vi "Cuadro de Texto.vi"(2 "Numeric":dbl, 3 "Read":refnum<k21>, 4 "Write":refnum<k21>, 5 "ECU TYPE":u16(ring) items=["LSMD", "LSMP", "LSMRL", "LSMRR"]) -> (0 "Write out":refnum<k21>, 1 "Read out":refnum<k21>)   [LabVIEW 2023]
panel:
  in  "OK":bool
  out "String":string
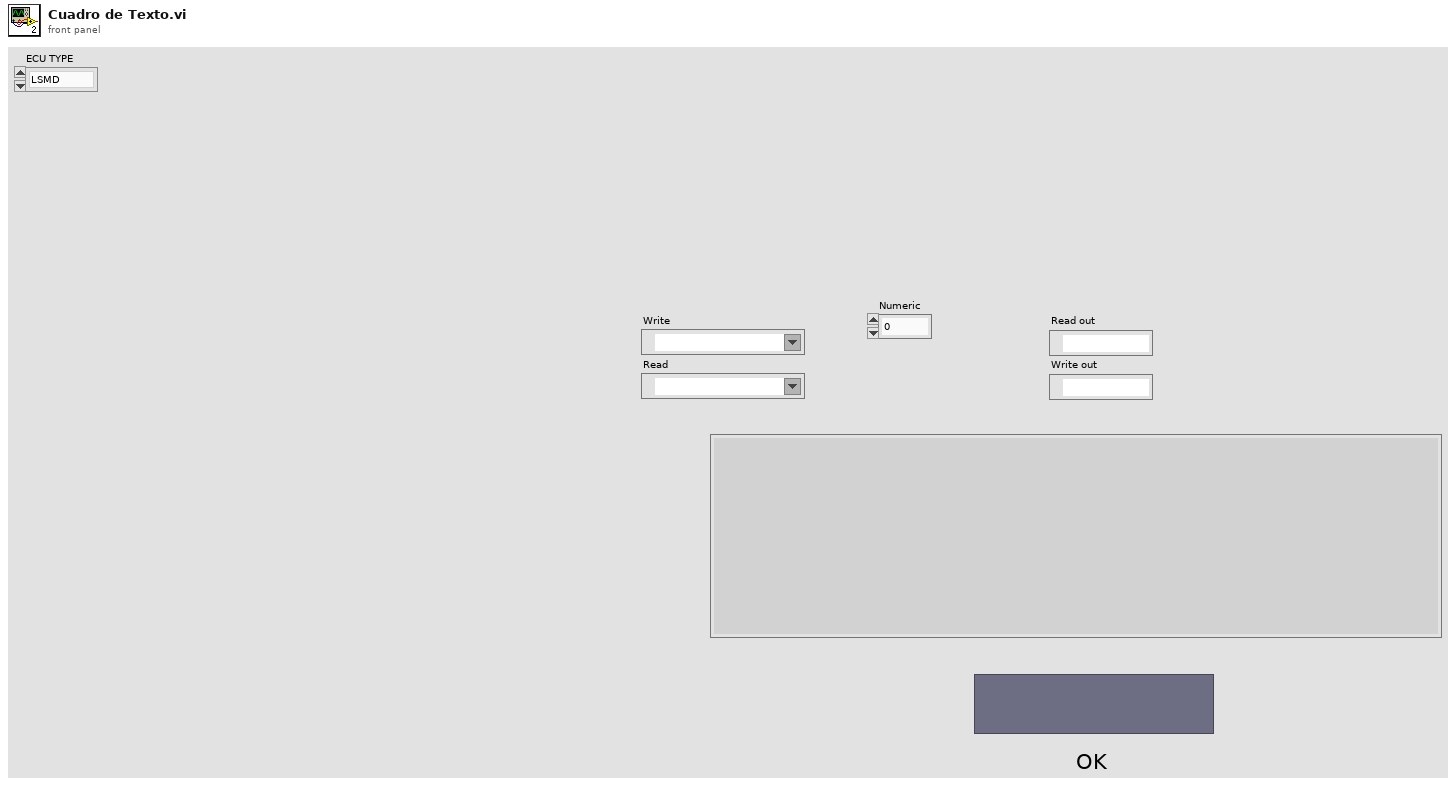
[diagram p1: front panel]
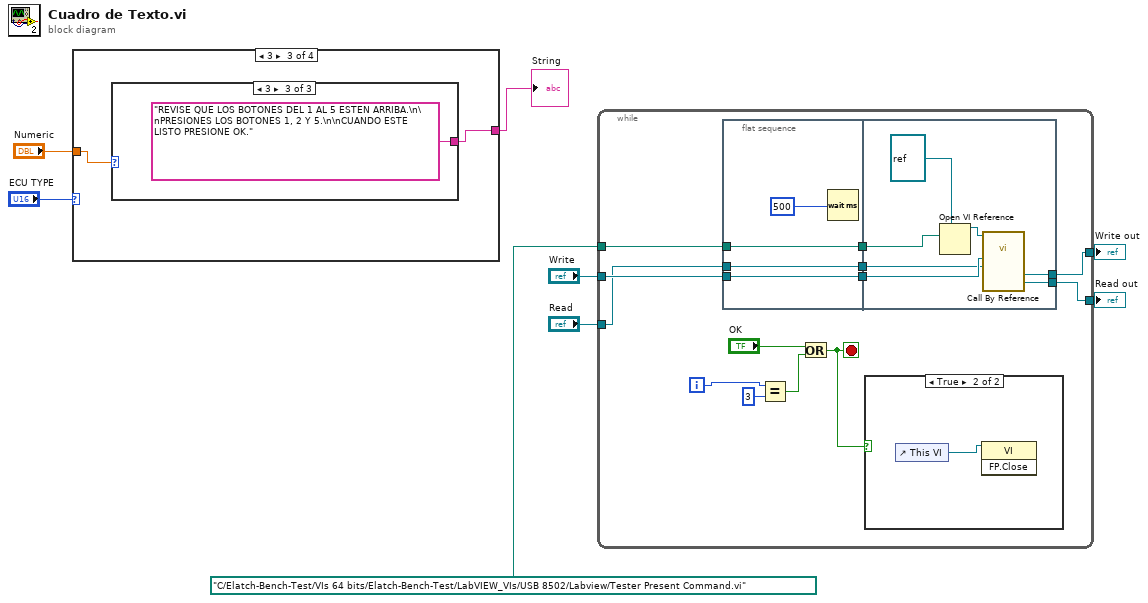
[diagram p0: block diagram]
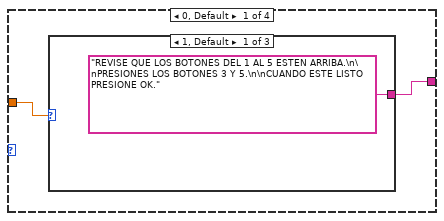
[diagram p3: hidden frame]
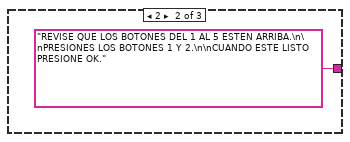
[diagram p4: hidden frame]
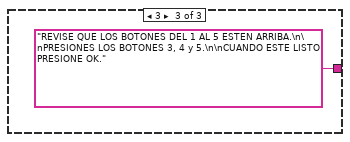
[diagram p5: hidden frame]
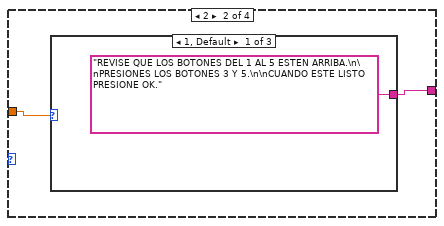
[diagram p6: hidden frame]
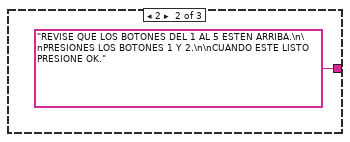
[diagram p7: hidden frame]
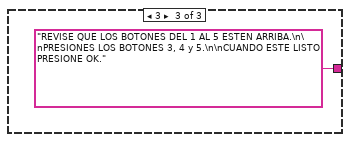
[diagram p8: hidden frame]
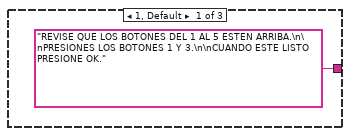
[diagram p9: hidden frame]
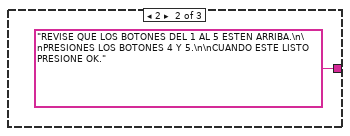
[diagram p10: hidden frame]
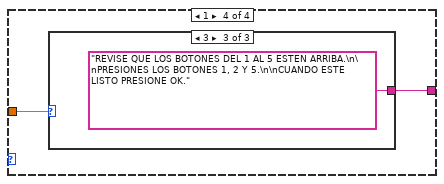
[diagram p11: hidden frame]
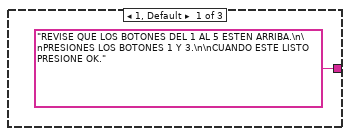
[diagram p12: hidden frame]
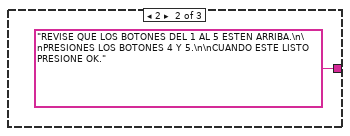
[diagram p13: hidden frame]
diagram:
  n1 = case shown="3" "ECU TYPE" {
    tunnel: "Numeric" -> [w10 w15 w20 w25]
    tunnel: [w9 w14 w19 w24] -> w1
    frame 0, Default {
      n2 = case shown="1, Default" w10 {
        tunnel: ["REVISE QUE LOS BOTONES DEL 1 AL 5 ESTEN ARRIBA.\n\nPRESIONES LOS BOTONES 3 Y 5.\n\nCUANDO ESTE LISTO PRESIONE OK." ("Message") "REVISE QUE LOS BOTONES DEL 1 AL 5 ESTEN ARRIBA.\n\nPRESIONES LOS BOTONES 1 Y 2.\n\nCUANDO ESTE LISTO PRESIONE OK." ("Message") "REVISE QUE LOS BOTONES DEL 1 AL 5 ESTEN ARRIBA.\n\nPRESIONES LOS BOTONES 3, 4 y 5.\n\nCUANDO ESTE LISTO PRESIONE OK." ("Message")] -> w9
        frame 1, Default {
        }
        frame 2 {
        }
        frame 3 {
        }
      }
    }
    frame 2 {
      n3 = case shown="1, Default" w15 {
        tunnel: ["REVISE QUE LOS BOTONES DEL 1 AL 5 ESTEN ARRIBA.\n\nPRESIONES LOS BOTONES 3 Y 5.\n\nCUANDO ESTE LISTO PRESIONE OK." ("Message") "REVISE QUE LOS BOTONES DEL 1 AL 5 ESTEN ARRIBA.\n\nPRESIONES LOS BOTONES 1 Y 2.\n\nCUANDO ESTE LISTO PRESIONE OK." ("Message") "REVISE QUE LOS BOTONES DEL 1 AL 5 ESTEN ARRIBA.\n\nPRESIONES LOS BOTONES 3, 4 y 5.\n\nCUANDO ESTE LISTO PRESIONE OK." ("Message")] -> w14
        frame 1, Default {
        }
        frame 2 {
        }
        frame 3 {
        }
      }
    }
    frame 3 {
      n4 = case shown="3" w20 {
        tunnel: ["REVISE QUE LOS BOTONES DEL 1 AL 5 ESTEN ARRIBA.\n\nPRESIONES LOS BOTONES 1 Y 3.\n\nCUANDO ESTE LISTO PRESIONE OK." ("Message") "REVISE QUE LOS BOTONES DEL 1 AL 5 ESTEN ARRIBA.\n\nPRESIONES LOS BOTONES 4 Y 5.\n\nCUANDO ESTE LISTO PRESIONE OK." ("Message") "REVISE QUE LOS BOTONES DEL 1 AL 5 ESTEN ARRIBA.\n\nPRESIONES LOS BOTONES 1, 2 Y 5.\n\nCUANDO ESTE LISTO PRESIONE OK." ("Message")] -> w19
        frame 1, Default {
        }
        frame 2 {
        }
        frame 3 {
        }
      }
    }
    frame 1 {
      n5 = case shown="3" w25 {
        tunnel: ["REVISE QUE LOS BOTONES DEL 1 AL 5 ESTEN ARRIBA.\n\nPRESIONES LOS BOTONES 1 Y 3.\n\nCUANDO ESTE LISTO PRESIONE OK." ("Message") "REVISE QUE LOS BOTONES DEL 1 AL 5 ESTEN ARRIBA.\n\nPRESIONES LOS BOTONES 4 Y 5.\n\nCUANDO ESTE LISTO PRESIONE OK." ("Message") "REVISE QUE LOS BOTONES DEL 1 AL 5 ESTEN ARRIBA.\n\nPRESIONES LOS BOTONES 1, 2 Y 5.\n\nCUANDO ESTE LISTO PRESIONE OK." ("Message")] -> w24
        frame 1, Default {
        }
        frame 2 {
        }
        frame 3 {
        }
      }
    }
  }
  "String" <- w1
  n6 = while {
    tunnel: "Read" -> [w34]
    tunnel: "Write" -> [w35]
    tunnel: path "C:/Elatch-Bench-Test/VIs 64 bits/Elatch-Bench-Test/LabVIEW_VIs/USB 8502/Labview/Tester Present Command.vi" ("vi path") -> [w33]
    tunnel: [w37] -> w3
    tunnel: [w36] -> w2
    i -> [w38]
    stop <- w32 stop-if-true
    n7 = flat-sequence {
      tunnel: w33 -> [w43]
      tunnel: w34 -> [w44]
      tunnel: w35 -> [w45]
      tunnel: [w45] -> w31
      tunnel: [w44] -> w30
      tunnel: [w43] -> w29
      tunnel: [w50] -> w37
      tunnel: [w49] -> w36
      tunnel: w31 -> [w48]
      tunnel: w30 -> [w47]
      tunnel: w29 -> [w46]
      frame #0 {
        n8 = Wait (ms)(milliseconds to wait=u32 500) -> ()  [unwired: 1 out]
      }
      frame #1 {
        n9 = Open VI Reference(type specifier VI Refnum (for type only)=refnum<vi> refnum, vi path=w46) -> (vi reference=w52:refnum<vi>)  [unwired: 4 in, 1 out]
        n10 = call-by-ref "?"(reference=w52, "Read"=w47, "Write"=w48) -> ("Read out"=w50:refnum<k21>, "Write out"=w49:refnum<k21>)  [unwired: 3 in, 4 out]
      }
    }
    n11 = Equal?(x=w38, y=3) -> (x = y?=w41:bool)
    n12 = Or(x="OK", y=w41) -> (x .or. y?=w32:bool)
    n13 = case shown="True" w32 {
      frame False {
      }
      frame True {
        n14 = control-ref of="This VI"() -> (w53:refnum<vi>)
        n15 = invoke class="VI" method="FP.Close"(reference=w53) -> ()  [unwired: 2 in, 3 out]
      }
    }
  }
  "Write out" <- w2
  "Read out" <- w3
